vi "BayesianGaussianMixture.vi"(8 "error in":errorcluster) -> (0 "error out":errorcluster, 3 "out":refnum<class "BayesianGaussianMixture.lvclass">)   [LabVIEW 2020]
doc: "Variational Bayesian estimation of a Gaussian mixture.\n\n This class allows to infer an approximate posterior distribution over the\n parameters of a Gaussian mixture distribution. The effective number of\n components can be inferred from the data.\n\n This class implements two types of prior for the weights distribution: a\n finite mixture model with Dirichlet distribution and an infinite mixture\n model with the Dirichlet Process. In practice Dirichlet Process inference\n algorithm is approximated and uses a truncated distribution with a fixed\n maximum number of components (called the Stick-breaking representation).\n The number of components actually used almost always depends on the data.\n\n .. versionadded:: 0.18\n\n Read more in the :ref:`User Guide <bgmm>`.\n\n Parameters\n ----------\n n_components : int, default=1\n The number of mixture components. Depending on the data and the value\n of the `weight_concentration_prior` the model can decide to not use\n all the components by setting some component `weights_` to values very\n close to zero. The number of effective components is therefore smaller\n than n_components.\n\n covariance_type : {'full', 'tied', 'diag', 'spherical'}, default='full'\n String describing the type of covariance parameters to use.\n Must be one of::\n\n 'full' (each component has its own general covariance matrix),\n 'tied' (all components share the same general covariance matrix),\n 'diag' (each component has its own diagonal covariance matrix),\n 'spherical' (each component has its own single variance).\n\n tol : float, default=1e-3\n The convergence threshold. EM iterations will stop when the\n lower bound average gain on the likelihood (of the training data with\n respect to the model) is below this threshold.\n\n reg_covar : float, default=1e-6\n Non-negative regularization added to the diagonal of covariance.\n Allows to assure that the covariance matrices are all positive.\n\n max_iter : int, default=100\n The number of EM iterations to perform.\n\n n_init : int, default=1\n The number of initializations to perform. The result with the highest\n lower bound value on the likelihood is kept.\n\n init_params : {'kmeans', 'random'}, default='kmeans'\n The method used to initialize the weights, the means and the\n covariances.\n Must be one of::\n\n 'kmeans' : responsibilities are initialized using kmeans.\n 'random' : responsibilities are initialized randomly.\n\n weight_concentration_prior_type : str, default='dirichlet_process'\n String describing the type of the weight concentration prior.\n Must be one of::\n\n 'dirichlet_process' (using the Stick-breaking representation),\n 'dirichlet_distribution' (can favor more uniform weights).\n\n weight_concentration_prior : float | None, default=None.\n The dirichlet concentration of each component on the weight\n distribution (Dirichlet). This is commonly called gamma in the\n literature. The higher concentration puts more mass in\n the center and will lead to more components being active, while a lower\n concentration parameter will lead to more mass at the edge of the\n mixture weights simplex. The value of the parameter must be greater\n than 0. If it is None, it's set to ``1. / n_components``.\n\n mean_precision_prior : float | None, default=None.\n The precision prior on the mean distribution (Gaussian).\n Controls the extent of where means can be placed. Larger\n values concentrate the cluster means around `mean_prior`.\n The value of the parameter must be greater than 0.\n If it is None, it is set to 1.\n\n mean_prior : array-like, shape (n_features,), default=None.\n The prior on the mean distribution (Gaussian).\n If it is None, it is set to the mean of X.\n\n degrees_of_freedom_prior : float | None, default=None.\n The prior of the number of degrees of freedom on the covariance\n distributions (Wishart). If it is None, it's set to `n_features`.\n\n covariance_prior : float or array-like, default=None.\n The prior on the covariance distribution (Wishart).\n If it is None, the emiprical covariance prior is initialized using the\n covariance of X. The shape depends on `covariance_type`::\n\n (n_features, n_features) if 'full',\n (n_features, n_features) if 'tied',\n (n_features) if 'diag',\n float if 'spherical'\n\n random_state : int, RandomState instance or None, default=None\n Controls the random seed given to the method chosen to initialize the\n parameters (see `init_params`).\n In addition, it controls the generation of random samples from the\n fitted distribution (see the method `sample`).\n Pass an int for reproducible output across multiple function calls.\n See :term:`Glossary <random_state>`.\n\n warm_start : bool, default=False\n If 'warm_start' is True, the solution of the last fitting is used as\n initialization for the next call of fit(). This can speed up\n convergence when fit is called several times on similar problems.\n See :term:`the Glossary <warm_start>`.\n\n verbose : int, default=0\n Enable verbose output. If 1 then it prints the current\n initialization and each iteration step. If greater than 1 then\n it prints also the log probability and the time needed\n for each step.\n\n verbose_interval : int, default=10\n Number of iteration done before the next print.\n\n Attributes\n ----------\n weights_ : array-like of shape (n_components,)\n The weights of each mixture components.\n\n means_ : array-like of shape (n_components, n_features)\n The mean of each mixture component.\n\n covariances_ : array-like\n The covariance of each mixture component.\n The shape depends on `covariance_type`::\n\n (n_components,) if 'spherical',\n (n_features, n_features) if 'tied',\n (n_components, n_features) if 'diag',\n (n_components, n_features, n_features) if 'full'\n\n precisions_ : array-like\n The precision matrices for each component in the mixture. A precision\n matrix is the inverse of a covariance matrix. A covariance matrix is\n symmetric positive definite so the mixture of Gaussian can be\n equivalently parameterized by the precision matrices. Storing the\n precision matrices instead of the covariance matrices makes it more\n efficient to compute the log-likelihood of new samples at test time.\n The shape depends on ``covariance_type``::\n\n (n_components,) if 'spherical',\n (n_features, n_features) if 'tied',\n (n_components, n_features) if 'diag',\n (n_components, n_features, n_features) if 'full'\n\n precisions_cholesky_ : array-like\n The cholesky decomposition of the precision matrices of each mixture\n component. A precision matrix is the inverse of a covariance matrix.\n A covariance matrix is symmetric positive definite so the mixture of\n Gaussian can be equivalently parameterized by the precision matrices.\n Storing the precision matrices instead of the covariance matrices makes\n it more efficient to compute the log-likelihood of new samples at test\n time. The shape depends on ``covariance_type``::\n\n (n_components,) if 'spherical',\n (n_features, n_features) if 'tied',\n (n_components, n_features) if 'diag',\n (n_components, n_features, n_features) if 'full'\n\n converged_ : bool\n True when convergence was reached in fit(), False otherwise.\n\n n_iter_ : int\n Number of step used by the best fit of inference to reach the\n convergence.\n\n lower_bound_ : float\n Lower bound value on the likelihood (of the training data with\n respect to the model) of the best fit of inference.\n\n weight_concentration_prior_ : tuple or float\n The dirichlet concentration of each component on the weight\n distribution (Dirichlet). The type depends on\n ``weight_concentration_prior_type``::\n\n (float, float) if 'dirichlet_process' (Beta parameters),\n float if 'dirichlet_distribution' (Dirichlet parameters).\n\n The higher concentration puts more mass in\n the center and will lead to more components being active, while a lower\n concentration parameter will lead to more mass at the edge of the\n simplex.\n\n weight_concentration_ : array-like of shape (n_components,)\n The dirichlet concentration of each component on the weight\n distribution (Dirichlet).\n\n mean_precision_prior_ : float\n The precision prior on the mean distribution (Gaussian).\n Controls the extent of where means can be placed.\n Larger values concentrate the cluster means around `mean_prior`.\n If mean_precision_prior is set to None, `mean_precision_prior_` is set\n to 1.\n\n mean_precision_ : array-like of shape (n_components,)\n The precision of each components on the mean distribution (Gaussian).\n\n mean_prior_ : array-like of shape (n_features,)\n The prior on the mean distribution (Gaussian).\n\n degrees_of_freedom_prior_ : float\n The prior of the number of degrees of freedom on the covariance\n distributions (Wishart).\n\n degrees_of_freedom_ : array-like of shape (n_components,)\n The number of degrees of freedom of each components in the model.\n\n covariance_prior_ : float or array-like\n The prior on the covariance distribution (Wishart).\n The shape depends on `covariance_type`::\n\n (n_features, n_features) if 'full',\n (n_features, n_features) if 'tied',\n (n_features) if 'diag',\n float if 'spherical'\n\n \nAvailable methods:\nFit\nFit Predict\nPredict\nPredict Proba\nSample\nScore\nScore Samples\nGet Attributes\nGet Params\nSet Params"
uses:
  BayesianGaussianMixture.lvclass
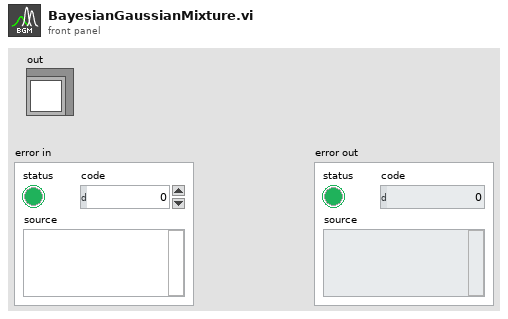
[diagram p1: front panel]
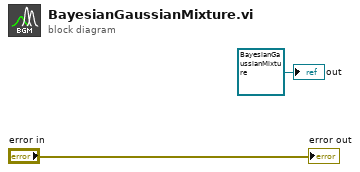
[diagram p0: block diagram]
diagram:
  "out" <- refnum<class "BayesianGaussianMixture.lvclass"> refnum ("model")
  "error out" <- "error in"
